vi "position_window.vi"() -> ()   [LabVIEW 2015]
uses:
  WINUTIL.LLB/Extract Window Origin / Size.vi
  global.vi
panel:
  out "Numeric":dbl
  out "centre y":dbl
  out "centre x":dbl
  out "offset y":dbl
  out "offset x":dbl
  # "how far away from the centre is the window?"
  # "where is the centre of the game window?"
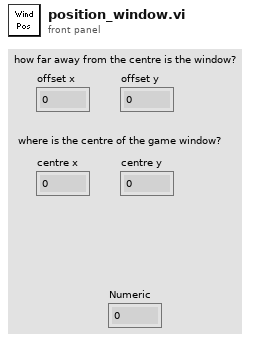
[diagram p1: front panel]
types:
  T1 = cluster{"Airspeed":dbl, "Altitude":dbl, "Vertical Speed":dbl, "Pitch":dbl, "Roll":dbl, "Heading":dbl, "Turn Indicator":dbl, "Latitude":dbl, "Longitude":dbl, "pilot g":dbl, "view number":i16, "fov":dbl, "view heading":dbl, "view pitch":dbl, "game width":i16, "game height":i16}
  T2 = typedef "Window Refnum" = refnum<k1>
  T3 = typedef "Window Rectangle.ctl" = cluster{"left":i16, "top":i16, "right":i16, "bottom":i16}
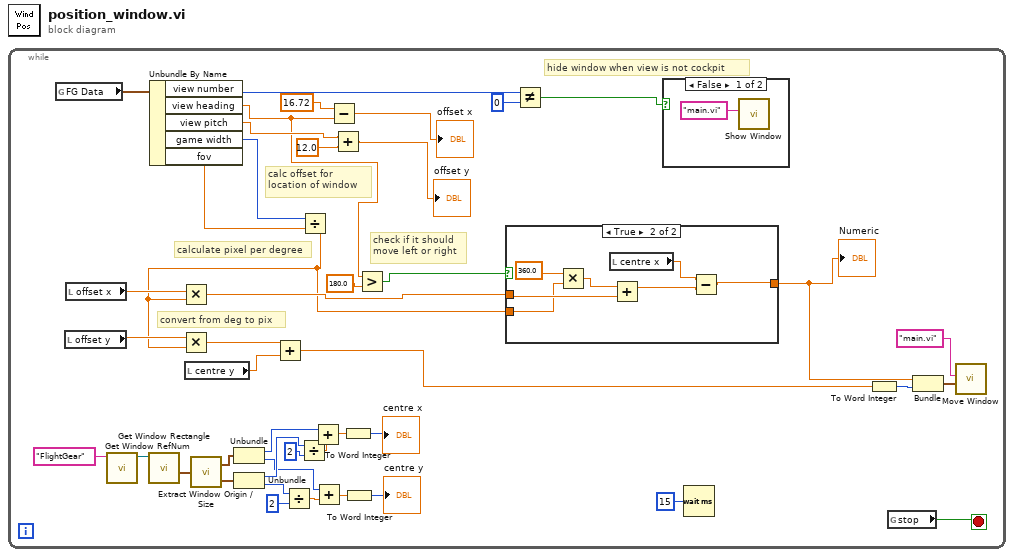
[diagram p0: block diagram]
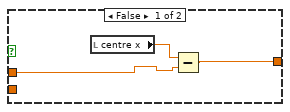
[diagram p2: hidden frame]
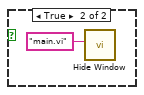
[diagram p3: hidden frame]
diagram:
  n1 = while {
    stop <- w1 stop-if-true
    # "check if it should\nmove left or right"
    # "convert from deg to pix"
    # "calc offset for \nlocation of window"
    # "calculate pixel per degree"
    # "hide window when view is not cockpit"
    n2 = global read "global.vi" "FG Data"() -> (w43:T1)
    n3 = local read "offset y"() -> (w29:dbl)
    n4 = local read "offset x"() -> (w30:dbl)
    n5 = call "Get Window RefNum.vi"("window name (\"\")"="FlightGear" ("window name (\"\")")) -> ("window refnum (NaWR)"=w39:T2)  [unwired: 7 in, 1 out]
    n6 = call "Get Window Rectangle.vi"("window refnum (NaWR)"=w39) -> ("window rect"=w37:T3)  [unwired: 4 in, 2 out]
    n7 = Unbundle By Name(w43) -> ("view number"=w41:i16, "view heading"=w7:dbl, "view pitch"=w15:dbl, "game width"=w34:i16, "fov"=w32:dbl)
    n8 = local read "centre y"() -> (w12:dbl)
    n9 = call "Extract Window Origin / Size.vi"("window rect"=w37) -> ("window origin"=w36:cluster{"left":i16, "top":i16}, "window size"=w35:cluster{"width":i16, "height":i16})
    n10 = Unbundle(w36) -> ("left"=w28:i16, "top"=w19:i16)
    n11 = Unbundle(w35) -> ("width"=w25:i16, "height"=w18:i16)
    n12 = Divide(x=w18, y=i16 2) -> (x/y=w20:dbl)
    n13 = Divide(x=w25, y=i16 2) -> (x/y=w27:dbl)
    n14 = Divide(x=w34, y=w32) -> (x/y=w2:dbl)
    n15 = Multiply(x=w30, y=w2) -> (x*y=w4:dbl)
    n16 = Multiply(x=w29, y=w2) -> (x*y=w13:dbl)
    n17 = Add(x=w13, y=w12) -> (x+y=w9:dbl)
    n18 = Add(x=w28, y=w27) -> (x+y=w24:dbl)
    n19 = Add(x=w19, y=w20) -> (x+y=w21:dbl)
    n20 = Subtract(x=16.72 ("y"), y=w7) -> (x-y=→"offset x":dbl)
    n21 = Add(x=w15, y=12.0) -> (x+y=→"offset y":dbl)
    n22 = To Word Integer(number=w24) -> (16bit integer=→"centre x":i16)
    n23 = To Word Integer(number=w21) -> (16bit integer=→"centre y":i16)
    n24 = Greater?(x=w7, y=180.0) -> (0:w5:bool)
    n25 = case shown="True" w5 {
      tunnel: w4 -> [w45 w54]
      tunnel: [w47 w49] -> w3
      tunnel: w2 -> [_ w52]
      frame False {
        n26 = local read "centre x"() -> (w46:dbl)
        n27 = Subtract(x=w46, y=w45) -> (x-y=w47:dbl)
      }
      frame True {
        n28 = Multiply(x=360.0, y=w52) -> (x*y=w51:dbl)
        n29 = local read "centre x"() -> (w50:dbl)
        n30 = Add(x=w51, y=w54) -> (x+y=w48:dbl)
        n31 = Subtract(x=w50, y=w48) -> (x-y=w49:dbl)
      }
    }
    "Numeric" <- w3
    n32 = Not Equal?(x=w41, y=i16 0) -> (x != y?=w40:bool)
    n33 = case shown="False" w40 {
      frame False {
        n34 = call "Show Window.vi"("window name (\"\")"="main.vi" ("window name (\"\")")) -> ()  [unwired: 5 in, 2 out]
      }
      frame True {
        n35 = call "Hide Window.vi"("window name (\"\")"="main.vi" ("window name (\"\")")) -> ()  [unwired: 5 in, 2 out]
      }
    }
    n36 = Wait (ms)(milliseconds to wait=u32 15) -> ()  [unwired: 1 out]
    n37 = To Word Integer(number=w9) -> (16bit integer=w8:i16)
    n38 = global read "global.vi" "stop"() -> (w1:bool)
    n39 = Bundle(w3, w8) -> (w10:cluster{dbl, i16})  [unwired: 1 in]
    n40 = call "Move Window.vi"("new position (0,0)"=w10, "window name (\"\")"="main.vi" ("window name (\"\")")) -> ()  [unwired: 3 in, 3 out]
  }
